vi "LSMcontroller_v61_updatedROIselection.vi"() -> ()   [LabVIEW 2015] (continued)
                                n2129 = call "configuration.vi"("command"="get") -> ("config out"=w5014:T12)  [unwired: 2 in, 1 out]
                                n2130 = Unbundle By Name(w5014) -> ("LT timestamp"=w5013:u32)
                                n2131 = call "2pparameters.vi"("command"="get") -> ("params out"=w5018:T11)  [unwired: 1 in]
                                n2132 = in-place {
                                in-place-border: w5013 -> [w5022]
                                n2133 = in-place-cluster #42(w5018) -> ("aDO"=w5021:u32[])
                                n2134 = call "add channel to active arrayv2.vi"("line array in"=w5021, "line to add"=w5022) -> ("line array out"=w5020:u32[])  [unwired: 2 out]
                                n2135 = in-place-cluster #42("aDO"=w5020) -> (w5016:T11)
                                }
                                n2136 = call "2pparameters.vi"("Params in"=w5016, "command"="set") -> ()  [unwired: 1 out]
                                }
                                frame #1 {
                                n2137 = call "waveformparamsv2.vi"("command"="add DO", "add DO"=w5023) -> ()  [unwired: 3 in, 3 out]
                                }
                                frame #2 {
                                n2138 = call "waveformsDObuffer.vi"("command"="get") -> ("DO wf out"=w5028:digitalwaveform[])  [unwired: 1 in]
                                n2139 = Build Array (concatenate)(w5028, w5025) -> (w5027:digitalwaveform[])
                                n2140 = call "waveformsDObuffer.vi"("DO wf in"=w5027, "command"="set") -> ()  [unwired: 1 out]
                                }
                                }
                                }
                                frame 0 {
                                n2141 = stacked-sequence {
                                seq-local: [w5034 _ _] -> [_ w5044 w5061]
                                tunnel: w5033 -> [_ _ _]
                                tunnel: w5032 -> [_ _ _]
                                tunnel: w5031 -> [_ w5041 _]
                                tunnel: w5030 -> [_ _ w5060]
                                frame #0 {
                                n2142 = call "configuration.vi"("command"="get") -> ("config out"=w5039:T12)  [unwired: 2 in, 1 out]
                                n2143 = Unbundle By Name(w5039) -> ("LT timestamp"=w5035:u32)
                                n2144 = call "2pparameters.vi"("command"="get") -> ("params out"=w5038:T11)  [unwired: 1 in]
                                n2145 = Unbundle By Name(w5038) -> ("aDO"=w5036:u32[])
                                n2146 = Search 1D Array(1D array=w5036, element=w5035) -> (index of element=w5034:i32)  [unwired: 1 in]
                                }
                                frame #1 {
                                n2147 = local read "Measurement"() -> (w5043:T4)
                                n2148 = To Unsigned Long Integer(number=w5043) -> (unsigned 32bit integer=w5042:u32)
                                n2149 = case shown="5..7" w5042 {
                                tunnel: w5044 -> [_ w5048]
                                tunnel: w5041 -> [_ w5045]
                                frame 0..4, Default {
                                }
                                frame 5..7 {
                                n2150 = Index Array(array=w5045, index=0) -> (element=w5046:T19)
                                n2151 = call "waveformparamsv2.vi"("command"="get") -> ("Params out"=w5051:T15)  [unwired: 4 in, 2 out]
                                n2152 = in-place {
                                in-place-border: w5048 -> [w5055]
                                in-place-border: w5046 -> [w5053]
                                n2153 = in-place-cluster #43(w5051) -> ("DO parameters"=w5056:T18)
                                n2154 = in-place {
                                in-place-border: w5053 -> [w5057]
                                n2155 = in-place-array #44(w5056, w5055) -> ()  [unwired: 1 out]
                                n2156 = in-place-array #44(w5057) -> (w5054:T18)  [unwired: 1 out]
                                }
                                n2157 = in-place-cluster #43("DO parameters"=w5054) -> (w5049:T15)
                                }
                                n2158 = call "waveformparamsv2.vi"("command"="set", "Params in"=w5049) -> ()  [unwired: 3 in, 3 out]
                                }
                                }
                                }
                                frame #2 {
                                n2159 = local read "Measurement"() -> (w5059:T4)
                                n2160 = To Unsigned Long Integer(number=w5059) -> (unsigned 32bit integer=w5058:u32)
                                n2161 = case shown="5..7" w5058 {
                                tunnel: w5061 -> [_ w5065]
                                tunnel: w5060 -> [_ w5063]
                                frame 0..4, Default {
                                }
                                frame 5..7 {
                                n2162 = Index Array(array=w5063, index=0) -> (element=w5062:digitalwaveform)
                                n2163 = call "waveformsDObuffer.vi"("command"="get") -> ("DO wf out"=w5067:digitalwaveform[])  [unwired: 1 in]
                                n2164 = Replace Array Subset(array=w5067, new element=w5062, index=w5065) -> (w5069:digitalwaveform[])
                                n2165 = call "waveformsDObuffer.vi"("DO wf in"=w5069, "command"="set") -> ()  [unwired: 1 out]
                                }
                                }
                                }
                                }
                                }
                                }
                              }
                              frame #4 {
                                n2166 = call "Used AO lines.vi"() -> ("used AO names"=w5072:string[], "used AO lines"=w5070:tag[])  [unwired: 2 in]
                                n2167 = control-ref of="Analog Lines Plot"() -> (w5071:refnum<vi>)
                                n2168 = control-ref of="Digital Lines Plot"() -> (w5073:refnum<vi>)
                                n2169 = call "Used DO lines.vi"() -> ("used DO names"=w5074:string[], "used DO lines"=w5075:tag[])  [unwired: 2 in]
                                n2170 = local write "Analog Used Lines"(w5070) -> ()
                                n2171 = local write "Analog Used Names"(w5072) -> ()
                                n2172 = local write "Digital Used Lines"(w5075) -> ()
                                n2173 = local write "Digital Used Names"(w5074) -> ()
                                n2174 = call "prepDOWaveplot.vi"("DigitalGraph in"=w5073, "used DO names"=w5074) -> ()  [unwired: 1 in]
                                n2175 = call "prepAOWaveplot.vi"("WaveformGraph in"=w5071, "Analog Used Names"=w5072) -> ()  [unwired: 1 in]
                              }
                              frame #5 {
                                n2176 = local read "Meastab"() -> (w5090:enum32{"X-Y Image", "Linescan", "Timetrace"})
                                n2177 = property on="refwf" class="Ring (strict)"() -> ("RingText.Text"=w5087:string)  [unwired: 2 in, 2 out]
                                n2178 = case shown="\"Timetrace\"" w5090 {
                                tunnel: [w5092 w5093] -> w5091
                                frame "X-Y Image", Default {
                                n2179 = local read "Sampling rate"() -> (w5092:dbl)
                                }
                                frame "Timetrace" {
                                n2180 = local read "srateAODOtt"() -> (w5093:dbl)
                                }
                                }
                                n2181 = call "waveformsAObuffer.vi"("command"="get") -> ("AO wf out"=w5078:waveform(dbl)[])  [unwired: 1 in]
                                n2182 = local read "wavdet"() -> (w5088:bool)
                                n2183 = call "waveformsDObuffer.vi"("command"="get") -> ("DO wf out"=w5082:digitalwaveform[])  [unwired: 1 in]
                                n2184 = call "correctwaveformsizetemp.vi"("new sampling frequency (Hz)"=w5091, "start"=FALSE, "reference waveforms to"=w5087, "Analog waveforms in"=w5078, "stop"=TRUE, "Digital waveforms in"=w5082) -> ("analog wf out"=w5084:waveform(dbl)[], "Digital wf out"=w5086:digitalwaveform[], "measpoints"=w5089:i32)
                                n2185 = local write "Analog Lines Plot"(w5084) -> ()
                                n2186 = call "GetNumCamFramesv2.vi"("Digital Waveform Graph"=w5086) -> ("Numeric"=w5085:i32)  [unwired: 10 in]
                                n2187 = local write "Digital Lines Plot"(w5086) -> ()
                                n2188 = call "waveformsDObuffer.vi"("DO wf in"=w5086, "command"="set") -> ()  [unwired: 1 out]
                                n2189 = call "waveformsAObuffer.vi"("AO wf in"=w5084, "command"="set") -> ()  [unwired: 1 out]
                                n2190 = local write "Total Camera Frames"(w5085) -> ()
                                n2191 = case shown="True" w5088 {
                                tunnel: w5089 -> [_ w5094]
                                frame False {
                                }
                                frame True {
                                n2192 = local write "# of frames"(w5094) -> ()
                                }
                                }
                              }
                            }
                            n2193 = call "stoperaseCI.vi"() -> ()  [unwired: 12 in]
                            n2194 = call "stoperaseDO_img.vi"() -> ()  [unwired: 12 in]
                            n2195 = call "stoperaseAO_img.vi"() -> ()  [unwired: 12 in]
                            n2196 = call "stoperaseAI_img.vi"() -> ()  [unwired: 12 in]
                          }
                          frame #9 {
                            w5104 = FALSE ("Value (Signaling)")
                            n2197 = local read "save\ndata"() -> (w5099:bool)
                            n2198 = case shown="True" w5099 {
                              tunnel: w5098 -> [_ w5111]
                              frame False {
                              }
                              frame True {
                                n2199 = call "closebinaryfiles.vi"() -> ()  [unwired: 12 in]
                                n2200 = local read "filename prefix"() -> (w5113:string)
                                n2201 = local read "data dir"() -> (w5112:path)
                                n2202 = call "saveparams.vi"("timestamp"=w5111, "filename prefix in"=w5113, "data dir in"=w5112) -> ()  [unwired: 1 in]
                              }
                            }
                            n2203 = call "2pparameters.vi"("command"="get") -> ("params out"=w5095:T11)  [unwired: 1 in]
                            n2204 = Unbundle By Name(w5095) -> ("auto OD"=w5096:bool)
                            n2205 = case shown="True" w5096 {
                              frame False {
                              }
                              frame True {
                                n2206 = call "configuration.vi"("command"="get") -> ("config out"=w5107:T12)  [unwired: 2 in, 1 out]
                                n2207 = call "2pparameters.vi"("command"="get") -> ("params out"=w5110:T11)  [unwired: 1 in]
                                n2208 = Unbundle By Name(w5107) -> ("contour OD"=w5105:u16)
                                n2209 = Unbundle By Name(w5110) -> ("ODfilt"=w5106:u16)
                                n2210 = call "filterwheelcontrol_nothorlabslib.vi"("Current OD filt"=w5105, "New ODfilt"=w5106) -> ()  [unwired: 1 in]
                              }
                            }
                            n2211 = property on="Start" class="Bool (strict)"("Val(Sgnl)"=w5104) -> ()  [unwired: 2 in, 2 out]
                            n2212 = property on="Start" class="Bool (strict)"("Visible"=TRUE, "DisabledEnum"=T7."Enabled" ("Disabled")) -> ()  [unwired: 2 in, 2 out]
                            n2213 = property on="Stop" class="Bool (strict)"("Val(Sgnl)"=w5104) -> ()  [unwired: 2 in, 2 out]
                            n2214 = property on="Stop" class="Bool (strict)"("Visible"=FALSE, "DisabledEnum"=T7."Disabled" ("Disabled")) -> ()  [unwired: 2 in, 2 out]
                          }
                          frame #10 {
                            w5116 = T22 2 items=["no dialog", "OK message", "continue or stop message", "OK message + warnings", "continue/stop + warnings"] ("type of dialog (OK msg:1)")
                            n2215 = call "displayerrors.vi"() -> ("error IO"=w5117:errorcluster)
                            n2216 = call <vilib>:"General Error Handler.vi"("type of dialog (OK msg:1)"=w5116, "error in (no error)"=w5117) -> ("error out"=w5115:errorcluster)  [unwired: 9 in, 4 out]
                            n2217 = call <vilib>:"Clear Errors.vi"("error in (no error)"=w5115) -> ("error out"=w5114:errorcluster)  [unwired: 5 in, 1 out]
                            n2218 = call "seterrors.vi"("error IO"=w5114) -> ()
                          }
                        }
                      }
                    }
                  }
                  frame "Lifetime (point)" {
                    # "Disabled for conversion to 64 bit"
                    n2219 = disable-structure shown="Disabled" {
                      frame Disabled {
                        n2220 = stacked-sequence {
                          frame #0 {
                            w5128 = 12.5 ("x")
                            # "get from syncrate"
                            n2221 = local read "Bin size"() -> (w5122:T6)
                            n2222 = local read "Vx-ref"() -> (w5134:dbl)
                            n2223 = local read "Vy-ref"() -> (w5135:dbl)
                            n2224 = call "2pparameters.vi"("command"="get") -> ("params out"=w5120:T11)  [unwired: 1 in]
                            n2225 = Scale By Power Of 2(n=w5122, x=1.0 ("Y Scale.Range:Minimum")) -> (x*2^n=w5131:dbl)
                            n2226 = call "setposition.vi"("Vy"=w5135, "Vx"=w5134) -> ()  [unwired: 1 in]
                            n2227 = Unbundle By Name(w5120) -> ("autoshutter"=w5121:bool)
                            n2228 = Multiply(x=3000.0 ("Y Scale.Range:Minimum"), y=w5131) -> (x*y=w5129:dbl)
                            n2229 = Compound Arithmetic op=MULTIPLY(w5128, invert 3200.0 ("X Scale.Offset and Multiplier:Multiplier"), w5131) -> (w5130:dbl)
                            n2230 = case shown="True" w5121 {
                              frame False {
                              }
                              frame True {
                                n2231 = call "shuttercontrol.vi"("command"="open") -> ()  [unwired: 1 in, 1 out]
                              }
                            }
                            n2232 = call "lifetimeparameters.vi"("command"="get") -> ("Params out"=w5126:T20)  [unwired: 1 in]
                            n2233 = property on="Histogram" class="WFGraph (strict)"("XScale.Maximum"=w5128, "XScale.Minimum"=0.0 ("X Scale.Range:Minimum"), "YScale.Maximum"=w5129, "YScale.Minimum"=0.1 ("Y Scale.Range:Minimum"), "XScale.Multiplier"=w5130) -> ()  [unwired: 2 in, 2 out]
                            n2234 = Bundle By Name(cluster=w5126, "Bin size"=w5122) -> (w5127:T20)
                            n2235 = call "lifetimeparameters.vi"("Params in"=w5127, "command"="set") -> ()  [unwired: 1 out]
                            n2236 = property on="Histogram 2" class="WFGraph (strict)"("YScale.Maximum"=w5129, "XScale.Multiplier"=w5130, "XScale.Maximum"=w5128) -> ()  [unwired: 2 in, 2 out]
                            n2237 = call "2pparameters.vi"("command"="get") -> ("params out"=w5142:T11)  [unwired: 1 in]
                            n2238 = Bundle By Name(cluster=w5142, "type"="Lifetime (point)") -> (w5140:T11)
                            n2239 = property on="Stop" class="Bool (strict)"("Visible"=TRUE, "DisabledEnum"=T7."Enabled" ("Disabled")) -> ()  [unwired: 2 in, 2 out]
                            n2240 = property on="Start" class="Bool (strict)"("Visible"=FALSE, "DisabledEnum"=T7."Disabled and Grayed Out" ("Disabled")) -> ()  [unwired: 2 in, 2 out]
                            n2241 = call "2pparameters.vi"("Params in"=w5140, "command"="set") -> ()  [unwired: 1 out]
                          }
                          frame #1 {
                            n2242 = call "setup.vi"() -> ()  [unwired: 1 in]
                          }
                          frame #2 {
                            # "main loop"
                            n2243 = call "lifetimeparameters.vi"("command"="get") -> ("Params out"=w5152:T20)  [unwired: 1 in]
                            n2244 = Unbundle By Name(w5152) -> ("devidx"=w5150:i32)
                            n2245 = for {
                              N: 10000 -> [_]
                              tunnel: [w5153] -> w5148 mode=indexing
                              i -> [w5153]
                            }
                            n2246 = while {
                              tunnel: w5150 -> [w5157]
                              tunnel: w5148 -> [w5154]
                              i -> [w5155]
                              stop <- w5159 stop-if-true
                              n2247 = Increment(x=w5155) -> (x+1=w5156:i32)
                              n2248 = dll-call lib="phlib.dll" fn="_PH_GetCountRate@8" label="PH_GetCountRate"("devidx"=w5157, "channel"=0) -> (w5158:i32)  [unwired: 5 in, 2 out]
                              "SyncRate" <- w5158
                              n2249 = stacked-sequence {
                                seq-local: [_ _ w5166 _ _] -> [_ _ _ w5179 _]
                                seq-local: [_ _ w5165 _ _] -> [_ _ _ w5178 _]
                                seq-local: [_ w5163 _ _ _] -> [_ _ w5167 _ _]
                                tunnel: w5158 -> [_ _ _ w5186 _]
                                tunnel: w5154 -> [_ _ _ w5176 _]
                                frame #0 {
                                n2250 = call "start_binned.vi"() -> ()  [unwired: 1 in]
                                }
                                frame #1 {
                                n2251 = call "get-histogram.vi"() -> ("IntegralCount"=→"Integral count":u32, "Histogram"=w5163:u32[])
                                "Histogram" <- w5163
                                }
                                frame #2 {
                                n2252 = Search 1D Array(1D array=w5167, element=u32 0) -> (index of element=w5165:i32)  [unwired: 1 in]
                                n2253 = Multiply(x=w5165, y=0.99) -> (x*y=w5171:dbl)
                                n2254 = Array Subset(array=w5167, index=0, length=w5171) -> (w5174:u32[])
                                n2255 = Array Max & Min(array=w5174) -> (max index (indices)=w5168:i32)  [unwired: 3 out]
                                n2256 = Split 1D Array(array=w5174, index=w5168) -> (second subarray=w5170:u32[])  [unwired: 1 out]
                                n2257 = Array Max & Min(array=w5170) -> (min index (indices)=w5169:i32)  [unwired: 3 out]
                                n2258 = Split 1D Array(array=w5170, index=w5169) -> (first subarray=w5166:u32[])  [unwired: 1 out]
                                "Histogram 2" <- w5166
                                }
                                frame #3 {
                                n2259 = Array Size(array=w5179) -> (size(s)=w5181:i32)
                                n2260 = Array Subset(array=w5176, index=0, length=w5181) -> (w5180:i32[])
                                n2261 = Compound Arithmetic op=MULTIPLY(1000000000.0 ("value"), invert w5186, invert w5178, w5180) -> (w5177:dbl[])
                                n2262 = call <vilib>:"Exponential Fit.vi"("Y"=w5179, "X"=w5177) -> ("damping"=w5183:dbl)  [unwired: 8 in, 5 out]
                                n2263 = Divide(x=-1.0 ("y"), y=w5183) -> (x/y=→"Lifetime (ns)":dbl)
                                }
                                frame #4 {
                                n2264 = local read "downright"() -> (w5193:bool)
                                n2265 = local read "downleft"() -> (w5195:bool)
                                n2266 = local read "upright"() -> (w5191:bool)
                                n2267 = local read "upleft"() -> (w5189:bool)
                                n2268 = local read "down"() -> (w5194:bool)
                                n2269 = local read "right"() -> (w5192:bool)
                                n2270 = local read "left"() -> (w5196:bool)
                                n2271 = local read "up"() -> (w5190:bool)
                                n2272 = Compound Arithmetic op=OR(w5189, w5190, w5191, w5192, w5193, w5194, w5195, w5196) -> (w5188:bool)
                                n2273 = case shown="True" w5188 {
                                frame False {
                                }
                                frame True {
                                n2274 = stacked-sequence {
                                frame #0 {
                                n2275 = local read "downright"() -> (w5198:bool)
                                n2276 = local read "downleft"() -> (w5200:bool)
                                n2277 = local read "BigSmall"() -> (w5197:bool)
                                n2278 = local read "upright"() -> (w5202:bool)
                                n2279 = local read "upleft"() -> (w5205:bool)
                                n2280 = local read "down"() -> (w5201:bool)
                                n2281 = local read "right"() -> (w5203:bool)
                                n2282 = local read "left"() -> (w5199:bool)
                                n2283 = local read "up"() -> (w5204:bool)
                                n2284 = call "movestageparams.vi"("command"="get") -> ("Params out"=w5208:T21)  [unwired: 1 in]
                                n2285 = Bundle By Name(cluster=w5208, "upleft"=w5205, "up"=w5204, "upright"=w5202, "right"=w5203, "downright"=w5198, "down"=w5201, "downleft"=w5200, "left"=w5199, "Bigsmall"=w5197) -> (w5209:T21)
                                n2286 = call "movestageparams.vi"("Params in"=w5209, "command"="set") -> ()  [unwired: 1 out]
                                }
                                frame #1 {
                                n2287 = call "movestage.vi"() -> ()  [unwired: 12 in]
                                }
                                frame #2 {
                                w5210 = FALSE ("OK Button")
                                w5211 = FALSE ("OK Button")
                                n2288 = property on="down" class="Bool (strict)"("Value"=w5211) -> ()  [unwired: 2 in, 2 out]
                                n2289 = property on="up" class="Bool (strict)"("Value"=w5211) -> ()  [unwired: 2 in, 2 out]
                                n2290 = property on="right" class="Bool (strict)"("Value"=w5211) -> ()  [unwired: 2 in, 2 out]
                                n2291 = property on="left" class="Bool (strict)"("Value"=w5211) -> ()  [unwired: 2 in, 2 out]
                                n2292 = property on="upleft" class="Bool (strict)"("Value"=w5210) -> ()  [unwired: 2 in, 2 out]
                                n2293 = property on="upright" class="Bool (strict)"("Value"=w5210) -> ()  [unwired: 2 in, 2 out]
                                n2294 = property on="downleft" class="Bool (strict)"("Value"=w5210) -> ()  [unwired: 2 in, 2 out]
                                n2295 = property on="downright" class="Bool (strict)"("Value"=w5210) -> ()  [unwired: 2 in, 2 out]
                                }
                                }
                                }
                                }
                                }
                              }
                              n2296 = dll-call lib="phlib.dll" fn="_PH_GetCountRate@8" label="PH_GetCountRate"("devidx"=w5157, "channel"=1) -> (→"Ch1Rate":i32)  [unwired: 5 in, 2 out]
                              n2297 = local read "Stop"() -> (w5159:bool)
                              n2298 = local write "points recorded"(w5156) -> ()
                            }
                          }
                          frame #3 {
                            w5219 = FALSE ("Value (Signaling)")
                            n2299 = call "2pparameters.vi"("command"="get") -> ("params out"=w5213:T11)  [unwired: 1 in]
                            n2300 = Unbundle By Name(w5213) -> ("autoshutter"=w5214:bool)
                            n2301 = case shown="True" w5214 {
                              frame False {
                              }
                              frame True {
                                n2302 = call "shuttercontrol.vi"("command"="close") -> ()  [unwired: 1 in, 1 out]
                              }
                            }
                            n2303 = property on="Start" class="Bool (strict)"("Val(Sgnl)"=w5219) -> ()  [unwired: 2 in, 2 out]
                            n2304 = property on="Start" class="Bool (strict)"("Visible"=TRUE, "DisabledEnum"=T7."Enabled" ("Disabled")) -> ()  [unwired: 2 in, 2 out]
                            n2305 = property on="Stop" class="Bool (strict)"("Val(Sgnl)"=w5219) -> ()  [unwired: 2 in, 2 out]
                            n2306 = property on="Stop" class="Bool (strict)"("Visible"=FALSE, "DisabledEnum"=T7."Disabled" ("Disabled")) -> ()  [unwired: 2 in, 2 out]
                          }
                        }
                      }
                      frame Enabled {
                      }
                    }
                    n2307 = local write "64bit disabled"(TRUE ("64bit disabled")) -> ()
                  }
                }
              }
            }
          }
          event "avpp", "Angle ref", "xpixels ref", "Vx-min ref", "Vx-max ref", "ypixels ref", "Vy-min ref", "Vy-max ref", "ROI Type", "Sampling rate": Value Change {
            n2308 = event-data() -> ()  [unwired: 1 in, 6 out]
            n2309 = local read "avpp"() -> (w5238:i32)
            n2310 = local read "Angle ref"() -> (w5237:dbl)
            n2311 = local read "ROI Type"() -> (w5236:u16)
            n2312 = local read "xpixels ref"() -> (w5233:i32)
            n2313 = local read "Vx-min ref"() -> (w5232:dbl)
            n2314 = local read "Vx-max ref"() -> (w5231:dbl)
            n2315 = local read "ypixels ref"() -> (w5229:i32)
            n2316 = local read "Vy-min ref"() -> (w5230:dbl)
            n2317 = local read "Vy-max ref"() -> (w5226:dbl)
            n2318 = local read "Sampling rate"() -> (w5221:dbl)
            n2319 = local read "# of frames"() -> (w5225:i32)
            n2320 = local read "maxbufferAI"() -> (w5224:i32)
            n2321 = local read "Override AI buffer"() -> (w5222:bool)
            n2322 = call "2pparameters.vi"("command"="get") -> ("params out"=w5235:T11)  [unwired: 1 in]
            n2323 = Bundle By Name(cluster=w5235, "avpp"=w5238, "Angle Img"=w5237, "Xpixels Img"=w5233, "Vx-min Img"=w5232, "VX-max Img"=w5231, "Ypixels Img"=w5229, "Vy-min Img"=w5230, "Vy-max Img"=w5226, "srate"=w5221, "srate Img"=w5221, "measpoints"=w5225, "maxbufferAI"=w5224, "Drawing Mode"=w5236, "Vz-reset"=0.0, "AIoverride"=w5222) -> (w5227:T11)
            n2324 = call "2pparameters.vi"("Params in"=w5227, "command"="set") -> ()  [unwired: 1 out]
          }
          event "# of frames": Value Change {
            n2325 = event-data() -> ()  [unwired: 1 in, 6 out]
            n2326 = local read "Meastab"() -> (w5239:enum32{"X-Y Image", "Linescan", "Timetrace"})
            n2327 = case shown="\"X-Y Image\", Default" w5239 {
              frame "X-Y Image", Default {
                n2328 = local read "# of frames"() -> (w5240:i32)
                n2329 = call "2pparameters.vi"("command"="get") -> ("params out"=w5244:T11)  [unwired: 1 in]
                n2330 = Bundle By Name(cluster=w5244, "measpoints"=w5240) -> (w5241:T11)
                n2331 = call "2pparameters.vi"("Params in"=w5241, "command"="set") -> ()  [unwired: 1 out]
              }
              frame "Linescan" {
                n2332 = local read "srateAODOtt"() -> (w5254:dbl)
                n2333 = local read "# of frames"() -> (w5250:i32)
                n2334 = local read "refreshtime"() -> (w5256:dbl)
                n2335 = local read "bin"() -> (w5251:dbl)
                n2336 = call "tt_timeandsamples.vi"("bin"=w5251, "refreshtime"=w5256, "srateAODOtt"=w5254, "tot#ofsamples"=w5250) -> ("refreshrate"=w5253:dbl, "refreshbuffer"=w5252:i32, "timetracecycles"=w5249:i32)  [unwired: 5 in]
                n2337 = call "2pparameters.vi"("command"="get") -> ("params out"=w5246:T11)  [unwired: 1 in]
                n2338 = Bundle By Name(cluster=w5246, "measpoints"=w5250, "tt_cycles"=w5249, "refreshbuffer"=w5252, "refreshrate"=w5253) -> (w5248:T11)
                n2339 = Reciprocal(x=w5253) -> (1/x=w5255:dbl)
                n2340 = local write "refreshtime"(w5255) -> ()
                n2341 = call "2pparameters.vi"("Params in"=w5248, "command"="set") -> ()  [unwired: 1 out]
              }
              frame "Timetrace" {
                n2342 = local read "srateAODOtt"() -> (w5266:dbl)
                n2343 = local read "# of frames"() -> (w5262:i32)
                n2344 = local read "refreshtime"() -> (w5268:dbl)
                n2345 = local read "bin"() -> (w5263:dbl)
                n2346 = call "tt_timeandsamples.vi"("bin"=w5263, "refreshtime"=w5268, "srateAODOtt"=w5266, "tot#ofsamples"=w5262) -> ("refreshrate"=w5265:dbl, "refreshbuffer"=w5264:i32, "timetracecycles"=w5261:i32)  [unwired: 5 in]
                n2347 = call "2pparameters.vi"("command"="get") -> ("params out"=w5258:T11)  [unwired: 1 in]
                n2348 = Bundle By Name(cluster=w5258, "measpoints"=w5262, "tt_cycles"=w5261, "refreshbuffer"=w5264, "refreshrate"=w5265) -> (w5260:T11)
                n2349 = Reciprocal(x=w5265) -> (1/x=w5267:dbl)
                n2350 = local write "refreshtime"(w5267) -> ()
                n2351 = call "2pparameters.vi"("Params in"=w5260, "command"="set") -> ()  [unwired: 1 out]
              }
            }
          }
          event "srateAODOtt", "refreshtime", "Vx-ref", "Vy-ref", "Vx-min draw", "Vx-max draw", "Vy-min draw", "Vy-max draw", "bin": Value Change {
            n2352 = event-data() -> ()  [unwired: 1 in, 6 out]
            n2353 = local read "ypixels ref"() -> (w5300:i32)
            n2354 = local read "Vy-min draw"() -> (w5276:dbl)
            n2355 = local read "Vy-max draw"() -> (w5275:dbl)
            n2356 = local read "Vx-min draw"() -> (w5278:dbl)
            n2357 = local read "Vx-max draw"() -> (w5277:dbl)
            n2358 = local read "xpixels ref"() -> (w5274:i32)
            n2359 = local read "ROI Type"() -> (w5273:u16)
            n2360 = local read "Pel"() -> (w5272:dbl)
            n2361 = local read "srateAODOtt"() -> (w5282:dbl)
            n2362 = local read "# of frames"() -> (w5287:i32)
            n2363 = local read "refreshtime"() -> (w5280:dbl)
            n2364 = local read "bin"() -> (w5285:dbl)
            n2365 = local read "Override AI buffer"() -> (w5270:bool)
            n2366 = local read "finite samples"() -> (w5294:bool)
            n2367 = local read "srateAODOtt"() -> (w5269:dbl)
            n2368 = local read "srateAODOtt"() -> (w5288:dbl)
            n2369 = local read "continuous"() -> (w5293:bool)
            n2370 = local read "Angle ref"() -> (w5279:dbl)
            n2371 = local read "wavdet"() -> (w5295:bool)
            n2372 = local read "Vx-ref"() -> (w5290:dbl)
            n2373 = local read "Vy-ref"() -> (w5292:dbl)
            n2374 = local read "avpp"() -> (w5291:i32)
            n2375 = call "tt_timeandsamples.vi"("bin"=w5285, "refreshtime"=w5280, "srateAODOtt"=w5282, "tot#ofsamples"=w5287) -> ("refreshrate"=w5283:dbl, "refreshbuffer"=w5284:i32, "timetracecycles"=w5289:i32)  [unwired: 5 in]
            n2376 = local read "bin"() -> (w5286:dbl)
            n2377 = call "2pparameters.vi"("command"="get") -> ("params out"=w5298:T11)  [unwired: 1 in]
            n2378 = Bundle By Name(cluster=w5298, "Drawing Mode"=w5273, "measpoints"=w5287, "tt_cycles"=w5289, "refreshbuffer"=w5284, "refreshrate"=w5283, "Vx-ref"=w5290, "Vy-ref"=w5292, "srate"=w5269, "finite"=w5294, "cont"=w5293, "wavdet"=w5295, "avpp"=w5291, "srateAODO"=w5288, "bufferAI"=w5284, "bin"=w5286, "Angle Img"=w5279, "Vxminref"=w5278, "Vxmaxref"=w5277, "Vyminref"=w5276, "Vymaxref"=w5275, "Xpixels Img"=w5274, "Ypixels Img"=w5300, "Pel"=w5272, "Vz-reset"=0.0, "AIoverride"=w5270) -> (w5296:T11)
            n2379 = Reciprocal(x=w5283) -> (1/x=w5281:dbl)
            n2380 = local write "refreshtime"(w5281) -> ()
            n2381 = call "2pparameters.vi"("Params in"=w5296, "command"="set") -> ()  [unwired: 1 out]
          }
          event "Init": Value Change {
            # "Disabled for conversion to 64 bit"
            n2382 = event-data() -> ()  [unwired: 1 in, 6 out]
            n2383 = disable-structure shown="Disabled" {
              frame Disabled {
                n2384 = flat-sequence {
                  frame #0 {
                    n2385 = local read "Measurement"() -> (w5302:T4)
                    n2386 = case shown="\"Lifetime (scan)\", \"Lifetime (contour)\"" w5302 {
                      frame "X-Y-t movie", Default {
                      }
                      frame "Lifetime (point)" {
                        n2387 = stacked-sequence {
                          frame #0 {
                            n2388 = call "initialize.vi"("mode"=0) -> ()
                          }
                          frame #1 {
                            n2389 = call "calib.vi"() -> ()  [unwired: 1 in]
                          }
                        }
                      }
                      frame "Lifetime (scan)", "Lifetime (contour)" {
                        n2390 = stacked-sequence {
                          frame #0 {
                            n2391 = call "initialize.vi"("mode"=3) -> ()
                          }
                          frame #1 {
                            n2392 = call "calib.vi"() -> ()  [unwired: 1 in]
                          }
                        }
                      }
                    }
                  }
                  frame #1 {
                    n2393 = property on="Start" class="Bool (strict)"("Visible"=TRUE, "DisabledEnum"=T7."Enabled" ("Disabled")) -> ()  [unwired: 2 in, 2 out]
                    n2394 = property on="Init" class="Bool (strict)"("Visible"=FALSE, "DisabledEnum"=T7."Disabled and Grayed Out" ("Disabled"), "Value"=FALSE ("Init")) -> ()  [unwired: 2 in, 2 out]
                  }
                }
              }
              frame Enabled {
              }
            }
            n2395 = local write "64bit disabled"(TRUE ("64bit disabled")) -> ()
          }
          event "Measurement": Value Change {
            n2396 = event-data() -> ()  [unwired: 1 in, 5 out]
            n2397 = case shown="\"X-Y-t movie\"" "Measurement" {
              frame "X-Y-t movie" {
                w5312 = T7."Disabled" ("Disabled")
                w5311 = FALSE ("Visible")
                n2398 = call "2pparameters.vi"("command"="get") -> ("params out"=w5322:T11)  [unwired: 1 in]
                n2399 = local write "graphtab"(T5."image" ("graphtab")) -> ()
                n2400 = local write "Save tab"(enum32{"withsave", "withoutsave"}."withsave" ("Save tab")) -> ()
                n2401 = Bundle By Name(cluster=w5322, "type"="X-Y-t movie") -> (w5320:T11)
                n2402 = call "2pparameters.vi"("Params in"=w5320, "command"="set") -> ()  [unwired: 1 out]
                n2403 = property on="refreshtime" class="DigNum (strict)"("Visible"=FALSE, "DisabledEnum"=T7."Disabled and Grayed Out" ("Disabled")) -> ()  [unwired: 2 in, 2 out]
                n2404 = property on="ttt" class="Enum (strict)"("Visible"=FALSE) -> ()  [unwired: 2 in, 2 out]
                n2405 = property on="# of frames" class="DigNum (strict)"("DisabledEnum"=T7."Enabled" ("Disabled"), "Caption.Text"="# of frames") -> ()  [unwired: 2 in, 2 out]
                n2406 = property on="continuous" class="Bool (strict)"("Visible"=TRUE, "DisabledEnum"=T7."Enabled" ("Disabled")) -> ()  [unwired: 2 in, 2 out]
                n2407 = property on="finite samples" class="Bool (strict)"("Visible"=TRUE, "DisabledEnum"=T7."Enabled" ("Disabled")) -> ()  [unwired: 2 in, 2 out]
                n2408 = property on="avpp" class="DigNum (strict)"("Visible"=TRUE, "DisabledEnum"=T7."Enabled" ("Disabled")) -> ()  [unwired: 2 in, 2 out]
                n2409 = property on="srateAODOtt" class="DigNum (strict)"("Visible"=FALSE, "DisabledEnum"=T7."Disabled" ("Disabled")) -> ()  [unwired: 2 in, 2 out]
                n2410 = local write "save\ndata"(TRUE ("save\ndata")) -> ()
                n2411 = property on="finite samples" class="Bool (strict)"("Val(Sgnl)"=TRUE ("continuous for display")) -> ()  [unwired: 2 in, 2 out]
                n2412 = property on="continuous" class="Bool (strict)"("Value"=FALSE ("continuous for display")) -> ()  [unwired: 2 in, 2 out]
                n2413 = property on="Current Average" class="DigNum (strict)"("Visible"=TRUE, "DisabledEnum"=T7."Enabled" ("Disabled")) -> ()  [unwired: 2 in, 2 out]
                n2414 = property on="img_CH1" class="IntGraph (strict)"("ZScale.Maximum"=7.0 ("Z Scale.Range:Maximum")) -> ()  [unwired: 2 in, 2 out]
                n2415 = property on="Sampling rate" class="DigNum (strict)"("Visible"=TRUE, "DisabledEnum"=T7."Enabled" ("Disabled")) -> ()  [unwired: 2 in, 2 out]
                n2416 = property on="Pel" class="DigNum (strict)"("Visible"=w5311, "DisabledEnum"=w5312) -> ()  [unwired: 2 in, 2 out]
                n2417 = property on="bin" class="DigNum (strict)"("Visible"=w5311, "DisabledEnum"=w5312) -> ()  [unwired: 2 in, 2 out]
                "Meastab" <- enum32{"X-Y Image", "Linescan", "Timetrace"}."X-Y Image" ("Meastab")
                "Zscantab" <- enum32{"withzscan", "withoutzscan", "lifetime"}."withoutzscan" ("Zscantab")
              }
              frame "X-Y-Z stack" {
                w5344 = T7."Disabled" ("Disabled")
                w5343 = FALSE ("Visible")
                n2418 = call "2pparameters.vi"("command"="get") -> ("params out"=w5354:T11)  [unwired: 1 in]
                n2419 = call "2pparameters.vi"("command"="get") -> ("params out"=w5358:T11)  [unwired: 1 in]
                n2420 = Bundle By Name(cluster=w5354, "type"="X-Y-Z stack") -> (w5352:T11)
                n2421 = Unbundle By Name(w5358) -> ("motorref"=w5357:refnum<k7>)
                n2422 = call "2pparameters.vi"("Params in"=w5352, "command"="set") -> ()  [unwired: 1 out]
                n2423 = local write "Zscantab"(enum32{"withzscan", "withoutzscan", "lifetime"}."withzscan" ("Zscantab")) -> ()
                n2424 = local write "Meastab"(enum32{"X-Y Image", "Linescan", "Timetrace"}."X-Y Image" ("Meastab")) -> ()
                n2425 = invoke class="MG17Motor" method="GetPosition"(reference=w5357, "lChanID"=0, "pfPosition"=sgl 0.0) -> ("pfPosition"=w5369:sgl)  [unwired: 2 in, 4 out]
                n2426 = property on="refreshtime" class="DigNum (strict)"("Visible"=FALSE, "DisabledEnum"=T7."Disabled and Grayed Out" ("Disabled")) -> ()  [unwired: 2 in, 2 out]
                n2427 = property on="ttt" class="Enum (strict)"("Visible"=FALSE) -> ()  [unwired: 2 in, 2 out]
                n2428 = Multiply(x=w5369, y=1000.0) -> (x*y=w5368:dbl)
                n2429 = local write "Actual Z position"(w5368) -> ()
                n2430 = local write "Save tab"(enum32{"withsave", "withoutsave"}."withsave" ("Save tab")) -> ()
                n2431 = property on="finite samples" class="Bool (strict)"("Visible"=FALSE, "DisabledEnum"=T7."Disabled and Grayed Out" ("Disabled")) -> ()  [unwired: 2 in, 2 out]
                n2432 = property on="avpp" class="DigNum (strict)"("Visible"=TRUE, "DisabledEnum"=T7."Enabled" ("Disabled")) -> ()  [unwired: 2 in, 2 out]
                n2433 = property on="continuous" class="Bool (strict)"("Visible"=FALSE, "DisabledEnum"=T7."Disabled and Grayed Out" ("Disabled")) -> ()  [unwired: 2 in, 2 out]
                n2434 = property on="img_CH1" class="IntGraph (strict)"("ZScale.Maximum"=7.0 ("Z Scale.Range:Maximum")) -> ()  [unwired: 2 in, 2 out]
                n2435 = property on="srateAODOtt" class="DigNum (strict)"("Visible"=FALSE, "DisabledEnum"=T7."Disabled" ("Disabled")) -> ()  [unwired: 2 in, 2 out]
                n2436 = property on="Pel" class="DigNum (strict)"("Visible"=w5343, "DisabledEnum"=w5344) -> ()  [unwired: 2 in, 2 out]
                n2437 = property on="bin" class="DigNum (strict)"("Visible"=w5343, "DisabledEnum"=w5344) -> ()  [unwired: 2 in, 2 out]
                n2438 = property on="Current Average" class="DigNum (strict)"("Visible"=TRUE, "DisabledEnum"=T7."Enabled" ("Disabled")) -> ()  [unwired: 2 in, 2 out]
                n2439 = property on="# of frames" class="DigNum (strict)"("Caption.Text"="# of slices", "DisabledEnum"=T7."Disabled and Grayed Out" ("Disabled")) -> ()  [unwired: 2 in, 2 out]
                n2440 = local write "save\ndata"(TRUE ("save\ndata")) -> ()
                n2441 = property on="finite samples" class="Bool (strict)"("Val(Sgnl)"=TRUE ("continuous for display")) -> ()  [unwired: 2 in, 2 out]
                n2442 = property on="continuous" class="Bool (strict)"("Value"=FALSE ("continuous for display")) -> ()  [unwired: 2 in, 2 out]
                n2443 = property on="Sampling rate" class="DigNum (strict)"("Visible"=TRUE, "DisabledEnum"=T7."Enabled" ("Disabled")) -> ()  [unwired: 2 in, 2 out]
              }
              frame "X-Y-Z-t movie" {
                w5383 = T7."Disabled" ("Disabled")
                w5382 = FALSE ("Visible")
                n2444 = property on="# of frames" class="DigNum (strict)"("DisabledEnum"=T7."Enabled" ("Disabled")) -> ()  [unwired: 2 in, 2 out]
                n2445 = property on="Current Average" class="DigNum (strict)"("Visible"=TRUE, "DisabledEnum"=T7."Enabled" ("Disabled")) -> ()  [unwired: 2 in, 2 out]
                n2446 = property on="avpp" class="DigNum (strict)"("Visible"=TRUE, "DisabledEnum"=T7."Enabled" ("Disabled")) -> ()  [unwired: 2 in, 2 out]
                n2447 = local write "Save tab"(enum32{"withsave", "withoutsave"}."withsave" ("Save tab")) -> ()
                n2448 = local write "Zscantab"(enum32{"withzscan", "withoutzscan", "lifetime"}."withzscan" ("Zscantab")) -> ()
                n2449 = local write "Meastab"(enum32{"X-Y Image", "Linescan", "Timetrace"}."X-Y Image" ("Meastab")) -> ()
                n2450 = property on="refreshtime" class="DigNum (strict)"("Visible"=FALSE, "DisabledEnum"=T7."Disabled and Grayed Out" ("Disabled")) -> ()  [unwired: 2 in, 2 out]
                n2451 = property on="ttt" class="Enum (strict)"("Visible"=FALSE) -> ()  [unwired: 2 in, 2 out]
                n2452 = call "2pparameters.vi"("command"="get") -> ("params out"=w5393:T11)  [unwired: 1 in]
                n2453 = Bundle By Name(cluster=w5393, "type"="X-Y-Z-t movie") -> (w5391:T11)
                n2454 = property on="continuous" class="Bool (strict)"("Visible"=TRUE, "DisabledEnum"=T7."Enabled" ("Disabled")) -> ()  [unwired: 2 in, 2 out]
                n2455 = property on="finite samples" class="Bool (strict)"("Visible"=TRUE, "DisabledEnum"=T7."Enabled" ("Disabled")) -> ()  [unwired: 2 in, 2 out]
                n2456 = call "2pparameters.vi"("Params in"=w5391, "command"="set") -> ()  [unwired: 1 out]
                n2457 = property on="srateAODOtt" class="DigNum (strict)"("Visible"=FALSE, "DisabledEnum"=T7."Disabled" ("Disabled")) -> ()  [unwired: 2 in, 2 out]
                n2458 = local write "save\ndata"(TRUE ("save\ndata")) -> ()
                n2459 = property on="img_CH1" class="IntGraph (strict)"("ZScale.Maximum"=7.0 ("Z Scale.Range:Maximum")) -> ()  [unwired: 2 in, 2 out]
                n2460 = property on="continuous" class="Bool (strict)"("Value"=FALSE ("continuous for display")) -> ()  [unwired: 2 in, 2 out]
                n2461 = property on="finite samples" class="Bool (strict)"("Value"=TRUE ("continuous for display")) -> ()  [unwired: 2 in, 2 out]
                n2462 = property on="Sampling rate" class="DigNum (strict)"("Visible"=TRUE, "DisabledEnum"=T7."Enabled" ("Disabled")) -> ()  [unwired: 2 in, 2 out]
                n2463 = property on="Pel" class="DigNum (strict)"("Visible"=w5382, "DisabledEnum"=w5383) -> ()  [unwired: 2 in, 2 out]
                n2464 = property on="bin" class="DigNum (strict)"("Visible"=w5382, "DisabledEnum"=w5383) -> ()  [unwired: 2 in, 2 out]
              }
              frame "linescan" {
                w5413 = T7."Enabled" ("Disabled")
                w5412 = TRUE ("Visible")
                w5415 = T7."Enabled" ("Disabled")
                w5414 = TRUE ("Visible")
                n2465 = local write "Meastab"(enum32{"X-Y Image", "Linescan", "Timetrace"}."Linescan" ("Meastab")) -> ()
                n2466 = property on="Current Average" class="DigNum (strict)"("Visible"=TRUE, "DisabledEnum"=T7."Enabled" ("Disabled")) -> ()  [unwired: 2 in, 2 out]
                n2467 = local write "Save tab"(enum32{"withsave", "withoutsave"}."withsave" ("Save tab")) -> ()
                n2468 = local write "Zscantab"(enum32{"withzscan", "withoutzscan", "lifetime"}."withoutzscan" ("Zscantab")) -> ()
                n2469 = property on="refreshtime" class="DigNum (strict)"("Visible"=FALSE, "DisabledEnum"=T7."Disabled and Grayed Out" ("Disabled")) -> ()  [unwired: 2 in, 2 out]
                n2470 = property on="continuous" class="Bool (strict)"("Value"=FALSE ("continuous for display")) -> ()  [unwired: 2 in, 2 out]
                n2471 = property on="finite samples" class="Bool (strict)"("Value"=TRUE ("continuous for display")) -> ()  [unwired: 2 in, 2 out]
                n2472 = property on="ttt" class="Enum (strict)"("Visible"=FALSE) -> ()  [unwired: 2 in, 2 out]
                n2473 = local write "save\ndata"(TRUE ("save\ndata")) -> ()
                n2474 = call "2pparameters.vi"("command"="get") -> ("params out"=w5424:T11)  [unwired: 1 in]
                n2475 = Bundle By Name(cluster=w5424, "type"="linescan") -> (w5422:T11)
                n2476 = property on="# of frames" class="DigNum (strict)"("DisabledEnum"=T7."Enabled" ("Disabled"), "Caption.Text"="# of lines") -> ()  [unwired: 2 in, 2 out]
                n2477 = property on="continuous" class="Bool (strict)"("Visible"=TRUE, "DisabledEnum"=T7."Enabled" ("Disabled")) -> ()  [unwired: 2 in, 2 out]
                n2478 = property on="avpp" class="DigNum (strict)"("Visible"=TRUE, "DisabledEnum"=T7."Enabled" ("Disabled")) -> ()  [unwired: 2 in, 2 out]
                n2479 = property on="finite samples" class="Bool (strict)"("Visible"=TRUE, "DisabledEnum"=T7."Enabled" ("Disabled")) -> ()  [unwired: 2 in, 2 out]
                n2480 = property on="srateAODOtt" class="DigNum (strict)"("Visible"=TRUE, "DisabledEnum"=T7."Enabled" ("Disabled")) -> ()  [unwired: 2 in, 2 out]
                n2481 = call "2pparameters.vi"("Params in"=w5422, "command"="set") -> ()  [unwired: 1 out]
                n2482 = property on="Pel" class="DigNum (strict)"("Visible"=w5414, "DisabledEnum"=w5415) -> ()  [unwired: 2 in, 2 out]
                n2483 = property on="bin" class="DigNum (strict)"("Visible"=w5414, "DisabledEnum"=w5415) -> ()  [unwired: 2 in, 2 out]
                n2484 = property on="Sampling rate" class="DigNum (strict)"("Visible"=FALSE, "DisabledEnum"=T7."Disabled" ("Disabled")) -> ()  [unwired: 2 in, 2 out]
                n2485 = property on="Pel" class="DigNum (strict)"("Visible"=w5412, "DisabledEnum"=w5413) -> ()  [unwired: 2 in, 2 out]
                n2486 = property on="bin" class="DigNum (strict)"("Visible"=w5412, "DisabledEnum"=w5413) -> ()  [unwired: 2 in, 2 out]
              }
              frame "Timetrace" {
                w5445 = T7."Enabled" ("Disabled")
                w5444 = TRUE ("Visible")
                n2487 = call "2pparameters.vi"("command"="get") -> ("params out"=w5450:T11)  [unwired: 1 in]
                n2488 = local write "Meastab"(enum32{"X-Y Image", "Linescan", "Timetrace"}."Timetrace" ("Meastab")) -> ()
                n2489 = Unbundle By Name(w5450) -> ("Angle draw"=w5452:dbl)
                n2490 = local write "Zscantab"(enum32{"withzscan", "withoutzscan", "lifetime"}."withoutzscan" ("Zscantab")) -> ()
                n2491 = property on="# of frames" class="DigNum (strict)"("DisabledEnum"=T7."Enabled" ("Disabled"), "Caption.Text"="# of samples") -> ()  [unwired: 2 in, 2 out]
                n2492 = property on="refreshtime" class="DigNum (strict)"("Visible"=TRUE, "DisabledEnum"=T7."Enabled" ("Disabled")) -> ()  [unwired: 2 in, 2 out]
                n2493 = property on="avpp" class="DigNum (strict)"("Visible"=FALSE, "DisabledEnum"=T7."Disabled and Grayed Out" ("Disabled")) -> ()  [unwired: 2 in, 2 out]
                n2494 = property on="Current Average" class="DigNum (strict)"("Visible"=FALSE, "DisabledEnum"=T7."Disabled and Grayed Out" ("Disabled")) -> ()  [unwired: 2 in, 2 out]
                n2495 = local write "Angle drawing"(w5452) -> ()
                n2496 = property on="ttt" class="Enum (strict)"("Visible"=TRUE) -> ()  [unwired: 2 in, 2 out]
                n2497 = property on="continuous" class="Bool (strict)"("Visible"=TRUE, "DisabledEnum"=T7."Enabled" ("Disabled")) -> ()  [unwired: 2 in, 2 out]
                n2498 = property on="finite samples" class="Bool (strict)"("Visible"=TRUE, "DisabledEnum"=T7."Enabled" ("Disabled")) -> ()  [unwired: 2 in, 2 out]
                n2499 = local write "save\ndata"(TRUE ("save\ndata")) -> ()
                n2500 = property on="finite samples" class="Bool (strict)"("Val(Sgnl)"=TRUE ("continuous for display")) -> ()  [unwired: 2 in, 2 out]
                n2501 = property on="continuous" class="Bool (strict)"("Value"=FALSE ("continuous for display")) -> ()  [unwired: 2 in, 2 out]
                n2502 = local write "Save tab"(enum32{"withsave", "withoutsave"}."withsave" ("Save tab")) -> ()
                n2503 = property on="srateAODOtt" class="DigNum (strict)"("Visible"=TRUE, "DisabledEnum"=T7."Enabled" ("Disabled")) -> ()  [unwired: 2 in, 2 out]
                n2504 = call "2pparameters.vi"("command"="get") -> ("params out"=w5457:T11)  [unwired: 1 in]
                n2505 = Bundle By Name(cluster=w5457, "type"="Timetrace") -> (w5455:T11)
                n2506 = property on="Sampling rate" class="DigNum (strict)"("Visible"=FALSE, "DisabledEnum"=T7."Disabled" ("Disabled")) -> ()  [unwired: 2 in, 2 out]
                n2507 = property on="Pel" class="DigNum (strict)"("Visible"=w5444, "DisabledEnum"=w5445) -> ()  [unwired: 2 in, 2 out]
                n2508 = property on="bin" class="DigNum (strict)"("Visible"=w5444, "DisabledEnum"=w5445) -> ()  [unwired: 2 in, 2 out]
                n2509 = call "2pparameters.vi"("Params in"=w5455, "command"="set") -> ()  [unwired: 1 out]
              }
              frame "Lifetime (point)" {
                w5478 = T7."Enabled" ("Disabled")
                w5477 = TRUE ("Visible")
                n2510 = property on="Pel" class="DigNum (strict)"("Visible"=w5477, "DisabledEnum"=w5478) -> ()  [unwired: 2 in, 2 out]
                n2511 = property on="bin" class="DigNum (strict)"("Visible"=w5477, "DisabledEnum"=w5478) -> ()  [unwired: 2 in, 2 out]
                n2512 = property on="ttt" class="Enum (strict)"("Visible"=FALSE) -> ()  [unwired: 2 in, 2 out]
                n2513 = local write "Zscantab"(enum32{"withzscan", "withoutzscan", "lifetime"}."lifetime" ("Zscantab")) -> ()
                n2514 = local write "graphtab"(T5."Lifetime" ("graphtab")) -> ()
                n2515 = local write "Meastab"(enum32{"X-Y Image", "Linescan", "Timetrace"}."Timetrace" ("Meastab")) -> ()
                n2516 = call "lifetimeparameters.vi"("command"="get") -> ("Params out"=w5485:T20)  [unwired: 1 in]
                n2517 = Unbundle By Name(w5485) -> ("initialized"=w5486:bool)
                n2518 = property on="srateAODOtt" class="DigNum (strict)"("Visible"=TRUE, "DisabledEnum"=T7."Enabled" ("Disabled")) -> ()  [unwired: 2 in, 2 out]
                n2519 = case shown="False" w5486 {
                  frame False {
                    n2520 = property on="Init" class="Bool (strict)"("Visible"=TRUE, "DisabledEnum"=T7."Enabled" ("Disabled")) -> ()  [unwired: 2 in, 2 out]
                    n2521 = property on="Start" class="Bool (strict)"("Visible"=FALSE, "DisabledEnum"=T7."Disabled and Grayed Out" ("Disabled")) -> ()  [unwired: 2 in, 2 out]
                  }
                  frame True {
                  }
                }
                n2522 = property on="Sampling rate" class="DigNum (strict)"("Visible"=FALSE, "DisabledEnum"=T7."Disabled" ("Disabled")) -> ()  [unwired: 2 in, 2 out]
              }
              frame "Lifetime (scan)" {
                w5495 = T7."Disabled" ("Disabled")
                w5494 = FALSE ("Visible")
                n2523 = call "lifetimeparameters.vi"("command"="get") -> ("Params out"=w5507:T20)  [unwired: 1 in]
                n2524 = local write "graphtab"(T5."image" ("graphtab")) -> ()
                n2525 = local write "Save tab"(enum32{"withsave", "withoutsave"}."withsave" ("Save tab")) -> ()
                n2526 = local write "Meastab"(enum32{"X-Y Image", "Linescan", "Timetrace"}."X-Y Image" ("Meastab")) -> ()
                n2527 = local write "Zscantab"(enum32{"withzscan", "withoutzscan", "lifetime"}."lifetime" ("Zscantab")) -> ()
                n2528 = Unbundle By Name(w5507) -> ("initialized"=w5506:bool)
                n2529 = property on="ttt" class="Enum (strict)"("Visible"=FALSE) -> ()  [unwired: 2 in, 2 out]
                n2530 = property on="refreshtime" class="DigNum (strict)"("Visible"=FALSE, "DisabledEnum"=T7."Disabled and Grayed Out" ("Disabled")) -> ()  [unwired: 2 in, 2 out]
                n2531 = property on="Pel" class="DigNum (strict)"("Visible"=w5494, "DisabledEnum"=w5495) -> ()  [unwired: 2 in, 2 out]
                n2532 = property on="bin" class="DigNum (strict)"("Visible"=w5494, "DisabledEnum"=w5495) -> ()  [unwired: 2 in, 2 out]
                n2533 = property on="save data" class="Bool (strict)"("Visible"=TRUE, "DisabledEnum"=T7."Enabled" ("Disabled"), "Value"=TRUE ("Visible")) -> ()  [unwired: 2 in, 2 out]
                n2534 = case shown="False" w5506 {
                  frame False {
                    n2535 = property on="Init" class="Bool (strict)"("Visible"=TRUE, "DisabledEnum"=T7."Enabled" ("Disabled")) -> ()  [unwired: 2 in, 2 out]
                    n2536 = property on="Start" class="Bool (strict)"("Visible"=FALSE, "DisabledEnum"=T7."Disabled and Grayed Out" ("Disabled")) -> ()  [unwired: 2 in, 2 out]
                  }
                  frame True {
                  }
                }
                n2537 = call "2pparameters.vi"("command"="get") -> ("params out"=w5512:T11)  [unwired: 1 in]
                n2538 = property on="continuous" class="Bool (strict)"("Visible"=TRUE, "DisabledEnum"=T7."Disabled and Grayed Out" ("Disabled")) -> ()  [unwired: 2 in, 2 out]
                n2539 = property on="finite samples" class="Bool (strict)"("Visible"=TRUE, "DisabledEnum"=T7."Enabled" ("Disabled")) -> ()  [unwired: 2 in, 2 out]
                n2540 = Bundle By Name(cluster=w5512, "type"="Lifetime (scan)") -> (w5510:T11)
                n2541 = call "2pparameters.vi"("Params in"=w5510, "command"="set") -> ()  [unwired: 1 out]
                n2542 = property on="finite samples" class="Bool (strict)"("Val(Sgnl)"=TRUE ("continuous for display")) -> ()  [unwired: 2 in, 2 out]
                n2543 = property on="continuous" class="Bool (strict)"("Value"=FALSE ("continuous for display")) -> ()  [unwired: 2 in, 2 out]
                n2544 = property on="srateAODOtt" class="DigNum (strict)"("Visible"=FALSE, "DisabledEnum"=T7."Disabled" ("Disabled")) -> ()  [unwired: 2 in, 2 out]
                n2545 = property on="# of frames" class="DigNum (strict)"("DisabledEnum"=T7."Enabled" ("Disabled"), "Caption.Text"="# of frames") -> ()  [unwired: 2 in, 2 out]
                n2546 = property on="img_CH1" class="IntGraph (strict)"("ZScale.Maximum"=12.5 ("Z Scale.Range:Maximum")) -> ()  [unwired: 2 in, 2 out]
                n2547 = property on="Current Average" class="DigNum (strict)"("Visible"=TRUE, "DisabledEnum"=T7."Enabled" ("Disabled")) -> ()  [unwired: 2 in, 2 out]
                n2548 = property on="Sampling rate" class="DigNum (strict)"("Visible"=TRUE, "DisabledEnum"=T7."Enabled" ("Disabled")) -> ()  [unwired: 2 in, 2 out]
                n2549 = property on="avpp" class="DigNum (strict)"("Visible"=TRUE, "DisabledEnum"=T7."Enabled" ("Disabled")) -> ()  [unwired: 2 in, 2 out]
              }
              frame "Lifetime (contour)" {
                w5536 = T7."Enabled" ("Disabled")
                w5535 = TRUE ("Visible")
                n2550 = call "2pparameters.vi"("command"="get") -> ("params out"=w5543:T11)  [unwired: 1 in]
                n2551 = property on="# of frames" class="DigNum (strict)"("DisabledEnum"=T7."Enabled" ("Disabled"), "Caption.Text"="# of samples") -> ()  [unwired: 2 in, 2 out]
                n2552 = property on="refreshtime" class="DigNum (strict)"("Visible"=TRUE, "DisabledEnum"=T7."Enabled" ("Disabled")) -> ()  [unwired: 2 in, 2 out]
                n2553 = Unbundle By Name(w5543) -> ("Angle draw"=w5545:dbl)
                n2554 = property on="avpp" class="DigNum (strict)"("Visible"=FALSE, "DisabledEnum"=T7."Disabled and Grayed Out" ("Disabled")) -> ()  [unwired: 2 in, 2 out]
                n2555 = property on="Current Average" class="DigNum (strict)"("Visible"=FALSE, "DisabledEnum"=T7."Disabled and Grayed Out" ("Disabled")) -> ()  [unwired: 2 in, 2 out]
                n2556 = local write "Angle drawing"(w5545) -> ()
                n2557 = local write "Save tab"(enum32{"withsave", "withoutsave"}."withsave" ("Save tab")) -> ()
                n2558 = local write "Zscantab"(enum32{"withzscan", "withoutzscan", "lifetime"}."lifetime" ("Zscantab")) -> ()
                n2559 = local write "graphtab"(T5."Lifetime" ("graphtab")) -> ()
                n2560 = local write "Meastab"(enum32{"X-Y Image", "Linescan", "Timetrace"}."Timetrace" ("Meastab")) -> ()
                n2561 = property on="ttt" class="Enum (strict)"("Visible"=TRUE) -> ()  [unwired: 2 in, 2 out]
                n2562 = call "lifetimeparameters.vi"("command"="get") -> ("Params out"=w5567:T20)  [unwired: 1 in]
                n2563 = property on="finite samples" class="Bool (strict)"("Val(Sgnl)"=TRUE ("continuous for display")) -> ()  [unwired: 2 in, 2 out]
                n2564 = local write "save\ndata"(TRUE ("save\ndata")) -> ()
                n2565 = Unbundle By Name(w5567) -> ("initialized"=w5568:bool)
                n2566 = property on="continuous" class="Bool (strict)"("Visible"=TRUE, "DisabledEnum"=T7."Enabled" ("Disabled")) -> ()  [unwired: 2 in, 2 out]
                n2567 = property on="finite samples" class="Bool (strict)"("Visible"=TRUE, "DisabledEnum"=T7."Enabled" ("Disabled")) -> ()  [unwired: 2 in, 2 out]
                n2568 = property on="Pel" class="DigNum (strict)"("Visible"=w5535, "DisabledEnum"=w5536) -> ()  [unwired: 2 in, 2 out]
                n2569 = property on="bin" class="DigNum (strict)"("Visible"=w5535, "DisabledEnum"=w5536) -> ()  [unwired: 2 in, 2 out]
                n2570 = property on="continuous" class="Bool (strict)"("Value"=FALSE ("continuous for display")) -> ()  [unwired: 2 in, 2 out]
                n2571 = case shown="False" w5568 {
                  frame False {
                    n2572 = property on="Init" class="Bool (strict)"("Visible"=TRUE, "DisabledEnum"=T7."Enabled" ("Disabled")) -> ()  [unwired: 2 in, 2 out]
                    n2573 = property on="Start" class="Bool (strict)"("Visible"=FALSE, "DisabledEnum"=T7."Disabled and Grayed Out" ("Disabled")) -> ()  [unwired: 2 in, 2 out]
                  }
                  frame True {
                  }
                }
                n2574 = property on="srateAODOtt" class="DigNum (strict)"("Visible"=TRUE, "DisabledEnum"=T7."Enabled" ("Disabled")) -> ()  [unwired: 2 in, 2 out]
                n2575 = call "2pparameters.vi"("command"="get") -> ("params out"=w5547:T11)  [unwired: 1 in]
                n2576 = Bundle By Name(cluster=w5547, "type"="Timetrace") -> (w5541:T11)
                n2577 = call "2pparameters.vi"("Params in"=w5541, "command"="set") -> ()  [unwired: 1 out]
                n2578 = property on="Sampling rate" class="DigNum (strict)"("Visible"=FALSE, "DisabledEnum"=T7."Disabled" ("Disabled")) -> ()  [unwired: 2 in, 2 out]
              }
            }
          }
          event "Laserpower \n(%)": Value Change {
            n2579 = event-data() -> ("OldVal"=w5576:dbl, "NewVal"=w5577:dbl)  [unwired: 1 in, 4 out]
            n2580 = Not Equal?(x=w5576, y=w5577) -> (x != y?=w5578:bool)
            n2581 = case shown="True" w5578 {
              tunnel: w5577 -> [_ w5580]
              frame False {
              }
              frame True {
                n2582 = local read "wavelength(nm)"() -> (w5581:dbl)
                n2583 = call "configuration.vi"("command"="get") -> ("config out"=w5585:T12)  [unwired: 2 in, 1 out]
                n2584 = call "pockelscellcalibration.vi"("l"=w5581, "T"=w5580) -> ("Vout"=w5579:dbl)
                n2585 = Unbundle By Name(w5585) -> ("Vto2P"=w5584:i32, "AOlines"=w5583:tag[])
                n2586 = property on="lpow" class="DigNum (strict)"("Value"=w5580) -> ()  [unwired: 2 in, 2 out]
                n2587 = local write "Vpockels"(w5579) -> ()
                n2588 = Index Array(array=w5583, index=w5584) -> (element=w5582:tag)
                n2589 = call-poly <vilib>:"DAQmx Create Virtual Channel.vi"("physical channels"=w5582) -> ("task out"=w5588:refnum<k21>, "error out"=w5587:errorcluster)  [unwired: 13 in]
                n2590 = call-poly <vilib>:"DAQmx Write.vi"("task/channels in"=w5588, "data"=w5579, "error in"=w5587) -> ("task out"=w5589:refnum<k21>, "error out"=w5590:errorcluster)  [unwired: 10 in, 1 out]
                n2591 = call <vilib>:"DAQmx Start Task.vi"("task/channels in"=w5589, "error in"=w5590) -> ("task out"=w5591:refnum<k21>, "error out"=w5592:errorcluster)  [unwired: 12 in]
                n2592 = call <vilib>:"DAQmx Stop Task.vi"("task/channels in"=w5591, "error in"=w5592) -> ("task out"=w5593:refnum<k21>, "error out"=w5594:errorcluster)  [unwired: 12 in]
                n2593 = call <vilib>:"DAQmx Clear Task.vi"("task in"=w5593, "error in"=w5594) -> ()  [unwired: 13 in, 1 out]
              }
            }
          }
          event "lpow": Value Change {
            n2594 = event-data() -> ("OldVal"=w5595:dbl, "NewVal"=w5596:dbl)  [unwired: 1 in, 4 out]
            n2595 = Not Equal?(x=w5595, y=w5596) -> (x != y?=w5597:bool)
            n2596 = case shown="True" w5597 {
              tunnel: w5596 -> [_ w5600]
              frame False {
              }
              frame True {
                n2597 = local read "wavelength(nm)"() -> (w5599:dbl)
